vi "Send String.vi"(6 "FCT":u8, 7 "MAMP 2":u16, 8 "error in (no error)":errorcluster, 9 "SPM":u16, 10 "RES":u8=1, 11 "RAMP":u8=1) -> (0 "error out":errorcluster, 3 "Message":string)   [LabVIEW 2017]
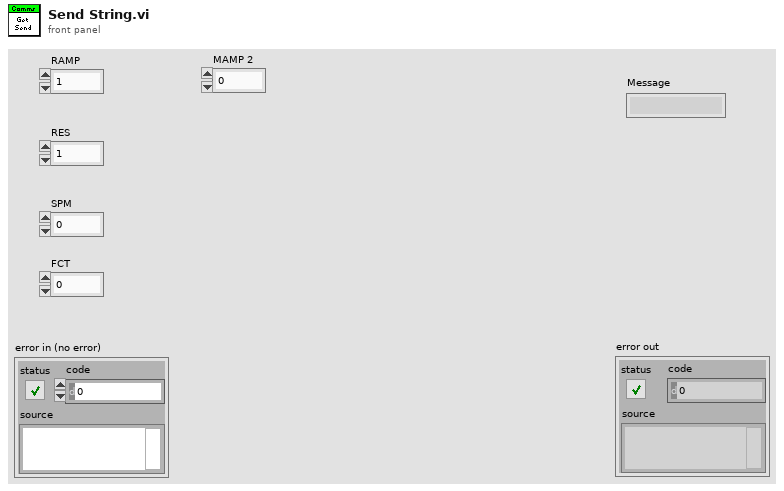
[diagram p1: front panel]
types:
  T1 = enum16{"Init", "Get Index", "Analyze Part", "Analyze Prts", "Analyze Prta", "Set VER", "Set TYPE"}
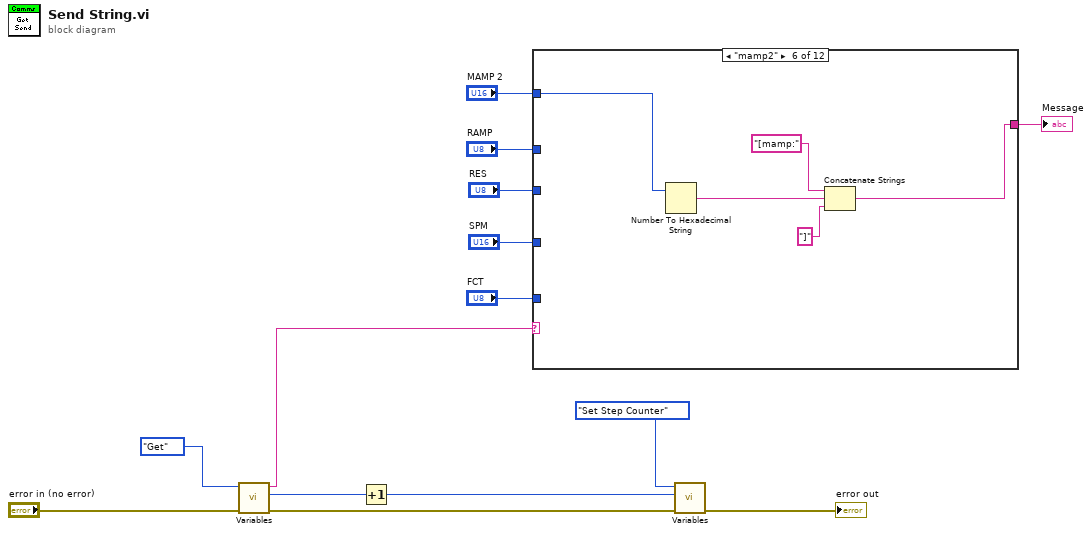
[diagram p0: block diagram]
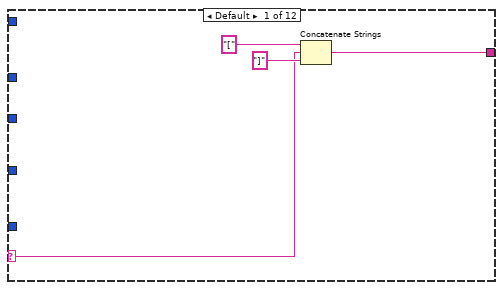
[diagram p2: hidden frame]
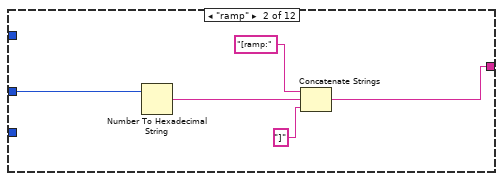
[diagram p3: hidden frame]
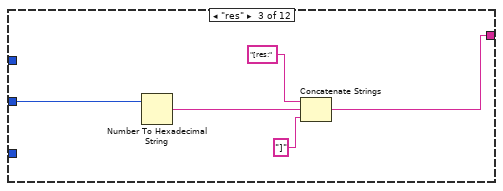
[diagram p4: hidden frame]
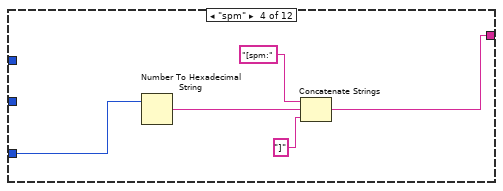
[diagram p5: hidden frame]
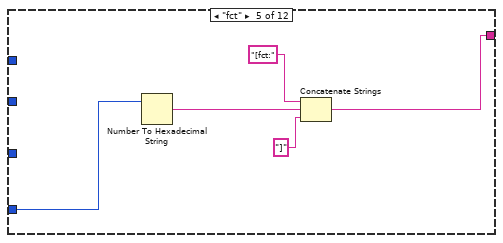
[diagram p6: hidden frame]
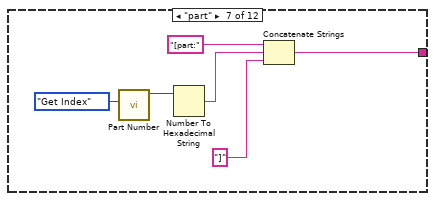
[diagram p7: hidden frame]
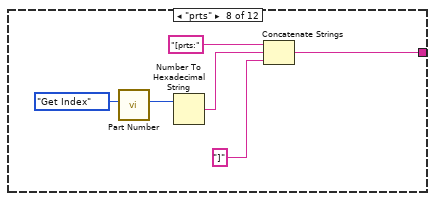
[diagram p8: hidden frame]
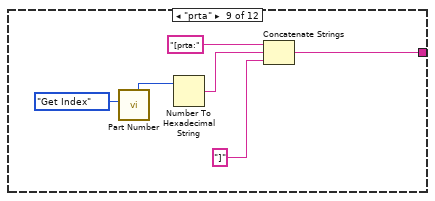
[diagram p9: hidden frame]
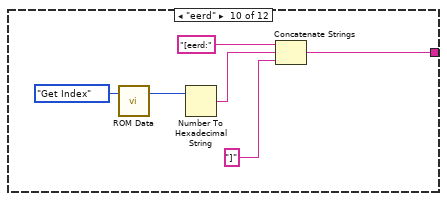
[diagram p10: hidden frame]
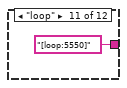
[diagram p11: hidden frame]
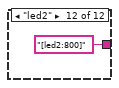
[diagram p12: hidden frame]
diagram:
  n1 = call "Variables.vi"("error in (no error)"="error in (no error)", "Command"=enum16{"Init", "Get", "Set Step Counter"}."Get") -> ("error out"=w11:errorcluster, "Step Counter"=w6:i32, "Out Message"=w4:string)  [unwired: 7 in]
  n2 = Increment(x=w6) -> (x+1=w5:i32)
  n3 = case shown="\"mamp2\"" w4 {
    selector: w4 -> [w16 _ _ _ _ _ _ _ _ _ _ _]
    tunnel: [w15 w20 w26 w31 w36 w41 w46 w52 w58 w64 "[loop:5550]" "[led2:800]"] -> w12
    tunnel: "RES" -> [_ _ w24 _ _ _ _ _ _ _ _ _]
    tunnel: "RAMP" -> [_ w23 _ _ _ _ _ _ _ _ _ _]
    tunnel: "SPM" -> [_ _ _ w29 _ _ _ _ _ _ _ _]
    tunnel: "FCT" -> [_ _ _ _ w34 _ _ _ _ _ _ _]
    tunnel: "MAMP 2" -> [_ _ _ _ _ w39 _ _ _ _ _ _]
    frame Default {
      n4 = Concatenate Strings("[" ("string"), w16, "]" ("string")) -> (w15:string)
    }
    frame "ramp" {
      n5 = Number To Hexadecimal String(2:w23) -> (0:w22:string)  [unwired: 1 in]
      n6 = Concatenate Strings("[ramp:", w22, "]" ("string")) -> (w20:string)
    }
    frame "res" {
      n7 = Number To Hexadecimal String(2:w24) -> (0:w28:string)  [unwired: 1 in]
      n8 = Concatenate Strings("[res:", w28, "]" ("string")) -> (w26:string)
    }
    frame "spm" {
      n9 = Number To Hexadecimal String(2:w29) -> (0:w33:string)  [unwired: 1 in]
      n10 = Concatenate Strings("[spm:", w33, "]" ("string")) -> (w31:string)
    }
    frame "fct" {
      n11 = Number To Hexadecimal String(2:w34) -> (0:w38:string)  [unwired: 1 in]
      n12 = Concatenate Strings("[fct:", w38, "]" ("string")) -> (w36:string)
    }
    frame "mamp2" {
      n13 = Number To Hexadecimal String(2:w39) -> (0:w43:string)  [unwired: 1 in]
      n14 = Concatenate Strings("[mamp:", w43, "]" ("string")) -> (w41:string)
    }
    frame "part" {
      n15 = call "Part Number.vi"("Command"=T1."Get Index") -> ("Part Index"=w45:i32)  [unwired: 5 in, 5 out]
      n16 = Number To Hexadecimal String(2:w45) -> (0:w48:string)  [unwired: 1 in]
      n17 = Concatenate Strings("[part:", w48, "]" ("string")) -> (w46:string)
    }
    frame "prts" {
      n18 = call "Part Number.vi"("Command"=T1."Get Index") -> ("Prts Index"=w51:i32)  [unwired: 5 in, 5 out]
      n19 = Number To Hexadecimal String(2:w51) -> (0:w54:string)  [unwired: 1 in]
      n20 = Concatenate Strings("[prts:", w54, "]" ("string")) -> (w52:string)
    }
    frame "prta" {
      n21 = call "Part Number.vi"("Command"=T1."Get Index") -> ("Prta Index"=w56:i32)  [unwired: 5 in, 5 out]
      n22 = Number To Hexadecimal String(2:w56) -> (0:w60:string)  [unwired: 1 in]
      n23 = Concatenate Strings("[prta:", w60, "]" ("string")) -> (w58:string)
    }
    frame "eerd" {
      n24 = call "ROM Data.vi"("Command"=enum16{"Init", "Get Index", "Analyze"}."Get Index") -> ("Index"=w63:i32)  [unwired: 1 in, 1 out]
      n25 = Number To Hexadecimal String(2:w63) -> (0:w66:string)  [unwired: 1 in]
      n26 = Concatenate Strings("[eerd:", w66, "]" ("string")) -> (w64:string)
    }
    frame "loop" {
    }
    frame "led2" {
    }
  }
  "Message" <- w12
  n27 = call "Variables.vi"("error in (no error)"=w11, "Value"=w5, "Command"=enum16{"Init", "Get", "Set Step Counter"}."Set Step Counter") -> ("error out"=→"error out":errorcluster)  [unwired: 6 in, 2 out]
